vi "time2.vi"() -> ()   [LabVIEW 2020]
panel:
  out "time 2":T1
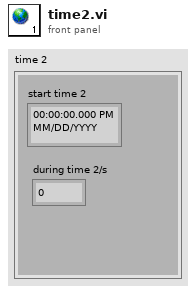
[diagram p1: front panel]
types:
  T1 = cluster{"start time 2":timestamp, "during time 2/s":dbl}
diagram:
